vi "test-slew-rate-limiter.vi"() -> (3 "All Tests Passed":bool)   [LabVIEW 2019]
uses:
  <vilib>/Rock Robotics/WPI/ThirdParty/JAS_Junk/TrajLib/SlewRateLimiter_New.vi
  <vilib>/Rock Robotics/WPI/ThirdParty/JAS_Junk/TrajLib/Util_GetTime.vi
  <vilib>/Rock Robotics/WPI/ThirdParty/JAS_Junk/TrajLib/Trajectory_Library.lvlib
panel:
  out "T1 = 0.5":dbl
  out "T0 -- < 2":dbl
  # "Slew Rate Limiter Test"
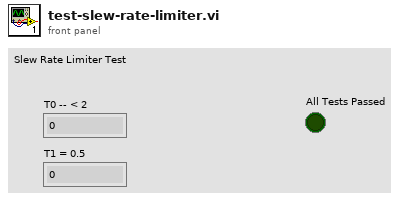
[diagram p1: front panel]
types:
  T1 = typedef "Trajectory_Library.lvlib/SLEW_RATE_LIMITER.ctl" = cluster{"RateLimit":dbl, "PrevValue":dbl, "PrevTime":dbl}
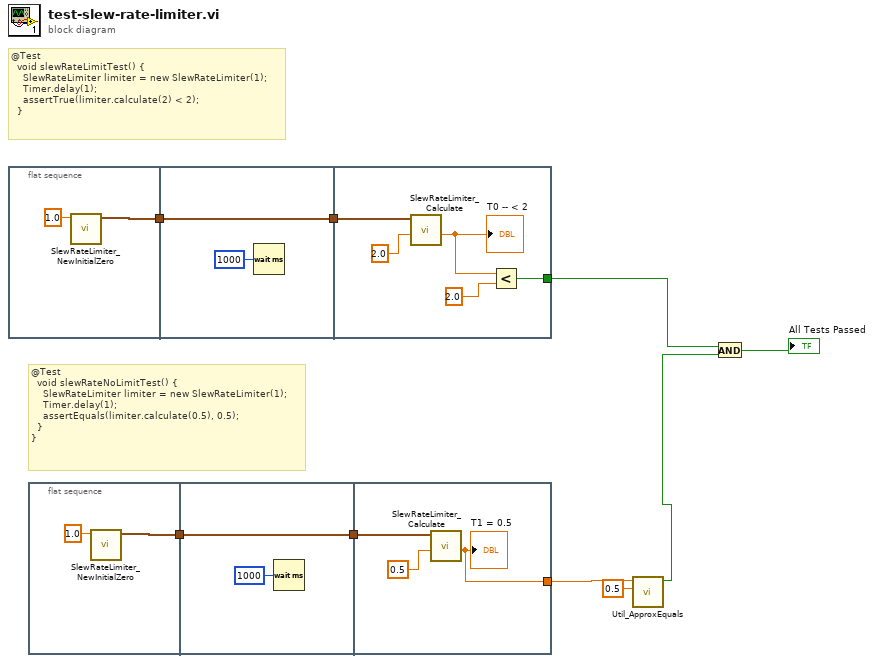
[diagram p0: block diagram]
diagram:
  # "@Test\n  void slewRateNoLimitTest() {\n    SlewRateLimiter limiter = new SlewRateLimiter(1);\n    Timer.delay(1);\n    assertEquals(limiter.calculate(0.5), 0.5);\n  }\n}"
  # "@Test\n  void slewRateLimitTest() {\n    SlewRateLimiter limiter = new SlewRateLimiter(1);\n    Timer.delay(1);\n    assertTrue(limiter.calculate(2) < 2);\n  }"
  n1 = flat-sequence {
    tunnel: [w10] -> w9
    tunnel: w9 -> [w12]
    tunnel: [w12] -> w8
    tunnel: w8 -> [w17]
    tunnel: [w14] -> w2
    frame #0 {
      n2 = call <vilib>:"SlewRateLimiter_NewInitialZero.vi"("RateLimit"=1.0) -> ("out SLEW_RATE_LIMITER"=w10:T1)  [unwired: 10 in]
    }
    frame #1 {
      n3 = Wait (ms)(milliseconds to wait=u32 1000) -> ()  [unwired: 1 out]
    }
    frame #2 {
      n4 = call <vilib>:"SlewRateLimiter_Calculate.vi"("Input"=2.0, "in SLEW_RATE_LIMITER"=w17) -> ("Output"=w16:dbl)  [unwired: 8 in, 1 out]
      "T0 -- < 2" <- w16
      n5 = Less?(x=w16, y=2.0) -> (x < y?=w14:bool)
    }
  }
  n6 = flat-sequence {
    tunnel: [w19] -> w7
    tunnel: w7 -> [w21]
    tunnel: [w21] -> w6
    tunnel: w6 -> [w24]
    tunnel: [w23] -> w5
    frame #0 {
      n7 = call <vilib>:"SlewRateLimiter_NewInitialZero.vi"("RateLimit"=1.0) -> ("out SLEW_RATE_LIMITER"=w19:T1)  [unwired: 10 in]
    }
    frame #1 {
      n8 = Wait (ms)(milliseconds to wait=u32 1000) -> ()  [unwired: 1 out]
    }
    frame #2 {
      n9 = call <vilib>:"SlewRateLimiter_Calculate.vi"("Input"=0.5, "in SLEW_RATE_LIMITER"=w24) -> ("Output"=w23:dbl)  [unwired: 8 in, 1 out]
      "T1 = 0.5" <- w23
    }
  }
  n10 = call <vilib>:"Util_ApproxEquals.vi"("Value 2"=0.5, "Value 1"=w5) -> ("ApproxEquals"=w3:bool)  [unwired: 9 in]
  n11 = And(x=w2, y=w3) -> (x .and. y?=→"All Tests Passed":bool)
